vi "write_FPGA_values.vi"(8 "error in (no error)":errorcluster, 10 "scan specification":T1={"x amplitude"=100, "x resolution (pixels)"=0, "x offset fly-forward (iterations)"=0, "x offset fly-back (iterations)"=100, "y resolution (nr. of lines)"=10, "y step size"=10, "iterations per pixel"=11, "number of frames"=0, "y offset (pixels)"=2, "number of y-brake lines  (before y-fly-back)"=2, "number y-brake lines (after y-fly-back)"=256, "number of y-fly-back steps"=8, "invert channel 0?"=FALSE, "invert channel 1?"=FALSE}, 11 "TrajectoryAK101022Resonance in":refnum<class "TrajectoryAK101022Resonance.lvclass">) -> (0 "error out":errorcluster, 3 "TrajectoryAK101022Resonance out":refnum<class "TrajectoryAK101022Resonance.lvclass">)   [LabVIEW 2010, in "TrajectoryAK101022Resonance.lvclass"]
uses:
  TrajectoryAK101022Resonance.lvclass
  FPGAWrapper/FPGAWrapperAK101022Resonance/scan_specification_cluster.ctl
  FPGAWrapper/FPGAWrapperAK101022Resonance/FPGAWrapperAK101022Resonance/FPGAWrapperAK101022Resonance.lvclass
  FPGAWrapper/GenericFPGAWrapper/GenericFPGAWrapper/GenericFPGAWrapper.lvclass
  TrajectoryAK101022Resonance.lvclass/TrajectoryAK101022Resonance.ctl
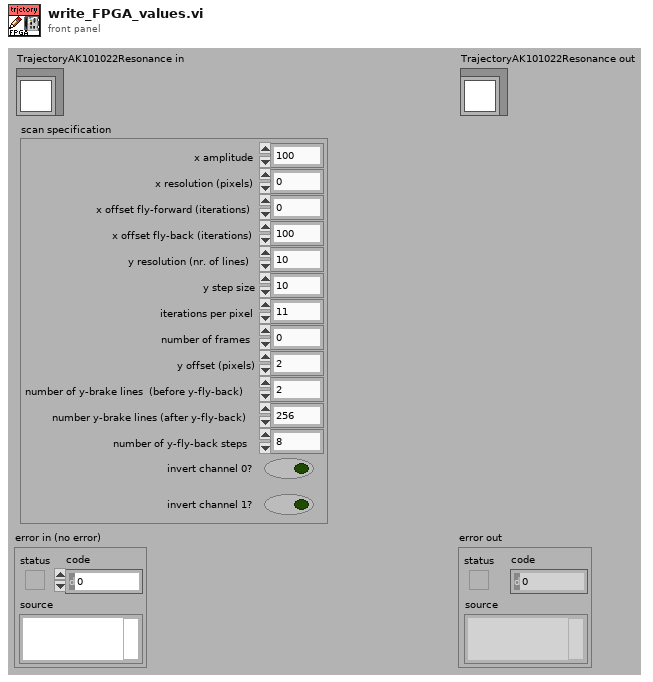
[diagram p1: front panel]
types:
  T1 = typedef "scan_specification_cluster.ctl" = cluster{"x amplitude":u16, "x resolution (pixels)":u16, "x offset fly-forward (iterations)":u16, "x offset fly-back (iterations)":u16, "y resolution (nr. of lines)":u16, "y step size":u16, "iterations per pixel":u16, "number of frames":i32, "y offset (pixels)":u16, "number of y-brake lines  (before y-fly-back)":u16, "number y-brake lines (after y-fly-back)":u16, "number of y-fly-back steps":u16, "invert channel 0?":bool, "invert channel 1?":bool}
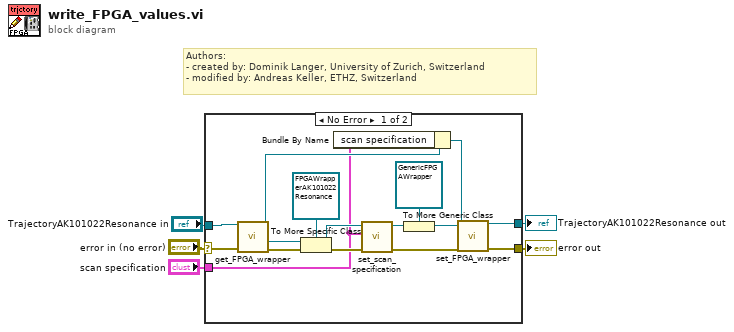
[diagram p0: block diagram]
diagram:
  # "Authors: \n- created by: Dominik Langer, University of Zurich, Switzerland\n- modified by: Andreas Keller, ETHZ, Switzerland"
  n1 = case shown="No Error" "error in (no error)" {
    selector: "error in (no error)" -> [w12 w23]
    tunnel: [w11 w23] -> w4
    tunnel: [w10 w22] -> w2
    tunnel: "TrajectoryAK101022Resonance in" -> [w13 w22]
    tunnel: "scan specification" -> [w7 _]
    frame No Error {
      n2 = call-dynamic "get_FPGA_wrapper.vi"("error in (no error)"=w12, "TrajectoryMG100122GenericFPGA in"=w13) -> ("error out"=w21:errorcluster, "GenericFPGAWrapper.lvclass"=w14:refnum<class "GenericFPGAWrapper.lvclass">, "TrajectoryMG100122GenericFPGA out"=w9:refnum<class "TrajectoryAK101022Resonance.lvclass">)  [unwired: 7 in]
      n3 = To More Specific Class(target class=refnum<class "FPGAWrapperAK101022Resonance.lvclass"> refnum ("FPGAWrapperAK101022Resonance.lvclass"), reference=w14, error in=w21) -> (specific class reference=w15:refnum<class "FPGAWrapperAK101022Resonance.lvclass">, error out=w20:errorcluster)
      n4 = Bundle By Name(cluster=w9, "scan specification"=w7) -> (w8:refnum<class "TrajectoryAK101022Resonance.lvclass">)
      n5 = call-dynamic "set_scan_specification.vi"("error in (no error)"=w20, "scan specification"=w7, "FPGA_AK101022Resonance in"=w15) -> ("error out"=w19:errorcluster, "FPGA_AK101022Resonance out"=w17:refnum<class "FPGAWrapperAK101022Resonance.lvclass">)  [unwired: 7 in]
      n6 = To More Generic Class(target class=refnum<class "GenericFPGAWrapper.lvclass"> refnum ("GenericFPGAWrapper.lvclass"), reference=w17) -> (generic class reference=w16:refnum<class "GenericFPGAWrapper.lvclass">)
      n7 = call-dynamic "set_FPGA_wrapper.vi"("error in (no error)"=w19, "GenericFPGAWrapper.lvclass"=w16, "TrajectoryMG100122GenericFPGA in"=w8) -> ("error out"=w11:errorcluster, "TrajectoryMG100122GenericFPGA out"=w10:refnum<class "TrajectoryAK101022Resonance.lvclass">)  [unwired: 7 in]
    }
    frame Error {
    }
  }
  "error out" <- w4
  "TrajectoryAK101022Resonance out" <- w2
